vi "DefaultFromIni.vi"(8 "error in (no error)":errorcluster, 11 "MyPluginsBase in":refnum<class "MyPluginsBase.lvclass">) -> (0 "error out":errorcluster, 3 "MyPluginsBase out":refnum<class "MyPluginsBase.lvclass">)   [LabVIEW 2014, in "MyPlugins.lvlib" / "MyPluginsBase.lvclass"]
doc: "This VI reads the ini file and performs any default configuration needed"
uses:
  MyPluginsBase.lvclass
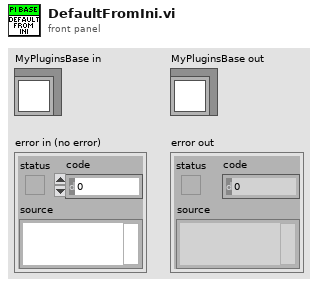
[diagram p1: front panel]
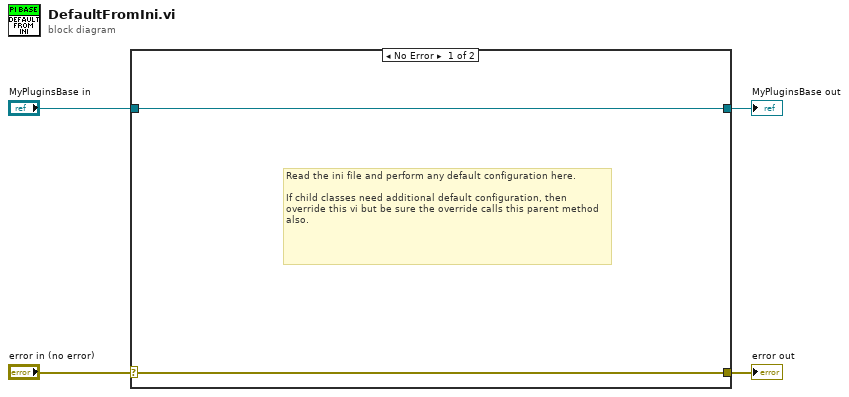
[diagram p0: block diagram]
diagram:
  n1 = case shown="No Error" "error in (no error)" {
    selector: "error in (no error)" -> [w5 w8]
    tunnel: [w5 w8] -> w3
    tunnel: [w6 w7] -> w1
    tunnel: "MyPluginsBase in" -> [w6 w7]
    frame No Error {
      # "Read the ini file and perform any default configuration here.\n\nIf child classes need additional default configuration, then override this vi but be sure the override calls this parent method also."
    }
    frame Error {
    }
  }
  "error out" <- w3
  "MyPluginsBase out" <- w1
